vi "Init Loop.vi"(8 "error in (no error)":errorcluster, 11 "HistorianCharting in":refnum<class "HistorianCharting.lvclass">) -> (0 "error out":errorcluster, 2 "Group Events":refnum<event-registration>, 3 "HistorianCharting out":refnum<class "HistorianCharting.lvclass">)   [LabVIEW 2020, in "VolatusGUIElements.lvlib" / "HistorianCharting.lvclass"]
uses:
  HistorianCharting.lvclass
  HistorianCharting.lvclass/HistorianCharting.ctl
  Volatus/VolatusAPI/VolatusAPI.lvclass
  VolatusGUI/Historian Charting Manager/X-Axis Type.ctl
  VolatusGUI/Historian Charting Manager/Historian Charting Manager.lvclass
  VolatusGUI/Historian Charting Manager/Scale.ctl
  VolatusGUI/Historian Charting Manager/Plot Config.ctl
  VolatusGUI/Historian Charting Manager/Plot Group Config.ctl
  VolatusGUI/Historian Charting Manager/Plot Group Changed Data.ctl
  VolatusGUI/Historian Charting Manager/Plot Group Removed Data.ctl
  VolatusGUI/Historian Charting Manager/New Plot Group Data.ctl
  VolatusGUI/Historian Charting Manager/Chart Select Group Data.ctl
  VolatusGUI/Historian Charting Manager/Plot Group Events.ctl
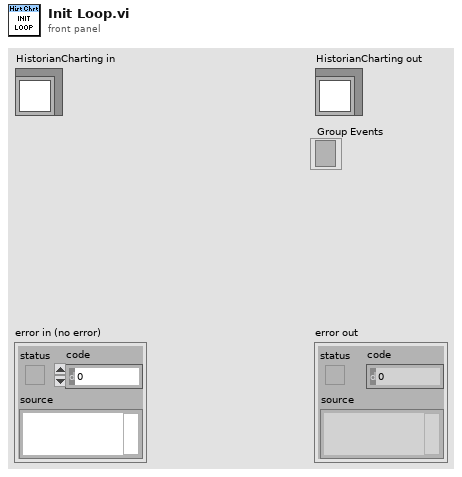
[diagram p1: front panel]
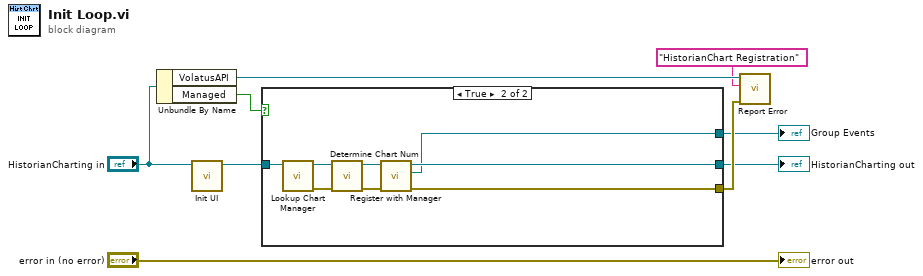
[diagram p0: block diagram]
diagram:
  n1 = Unbundle By Name("HistorianCharting in") -> ("VolatusAPI"=w4:refnum<class "VolatusAPI.lvclass">, "Managed"=w6:bool)
  n2 = call "Init UI.vi"("HistorianCharting in"="HistorianCharting in") -> ("HistorianCharting out"=w2:refnum<class "HistorianCharting.lvclass">)  [unwired: 9 in, 1 out]
  n3 = case shown="True" w6 {
    tunnel: w2 -> [w10 w18]
    tunnel: [w10 w13] -> w5
    tunnel: [_ w12] -> w9
    tunnel: [_ w11] -> w1
    frame False {
    }
    frame True {
      n4 = call "Lookup Chart Manager.vi"("HistorianCharting in"=w18) -> ("error out"=w16:errorcluster, "HistorianCharting out"=w17:refnum<class "HistorianCharting.lvclass">)  [unwired: 9 in]
      n5 = call "Determine Chart Num.vi"("error in (no error)"=w16, "HistorianCharting in"=w17) -> ("error out"=w15:errorcluster, "HistorianCharting out"=w14:refnum<class "HistorianCharting.lvclass">)  [unwired: 8 in]
      n6 = call "Register with Manager.vi"("error in (no error)"=w15, "HistorianCharting in"=w14) -> ("error out"=w12:errorcluster, "Group Events"=w11:refnum<event-registration>, "HistorianCharting out"=w13:refnum<class "HistorianCharting.lvclass">)  [unwired: 7 in]
    }
  }
  "HistorianCharting out" <- w5
  "Group Events" <- w1
  n7 = call "Report Error.vi"("error in (no error)"=w9, "Context"="HistorianChart Registration", "VolatusAPI in"=w4) -> ()  [unwired: 7 in, 2 out]
  "error out" <- "error in (no error)"
